vi "moveonapath.vi"() -> ()   [LabVIEW 2017]
uses:
  040-typeDefs/Position.ctl
panel:
  out "Waveform Chart":dbl(graph)
  in  "stop 2":bool
  out "XY Graph":cluster{"X":dbl, "Y":dbl}[](graph)
  in  "Array of Points":T1[](array[typedef])=[{"X Pos"=20.0, "Y Pos"=20.0, "Bearing"=0.0}]
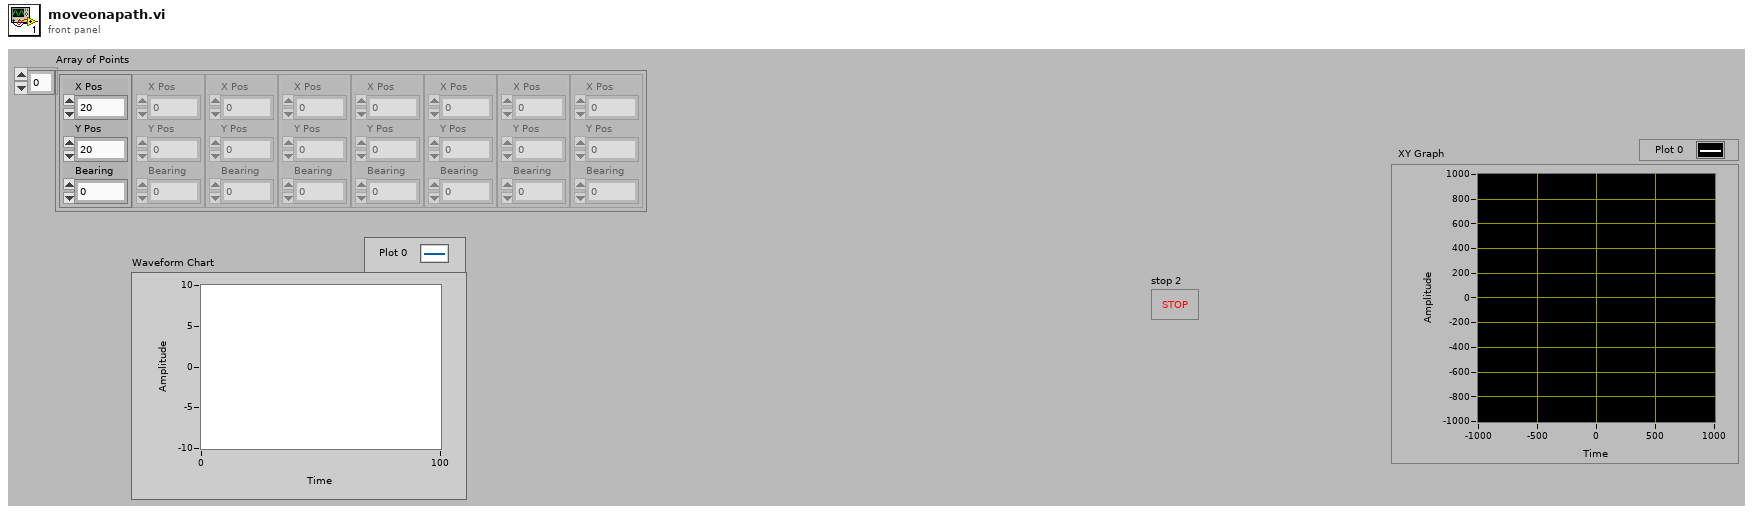
[diagram p1: front panel]
types:
  T1 = typedef "Position.ctl" = cluster{"X Pos":dbl, "Y Pos":dbl, "Bearing":dbl}
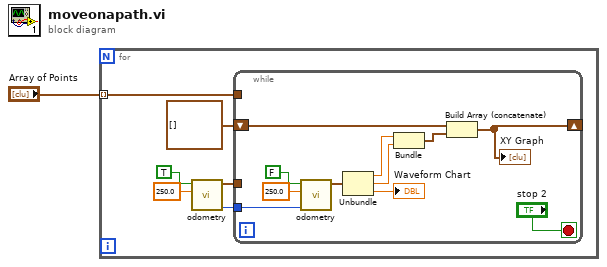
[diagram p0: block diagram]
diagram:
  n1 = for {
    tunnel: "Array of Points" -> [w2] mode=indexing
    n2 = call "odometry.vi"("wheelbase"=250.0, "Position"=TRUE) -> ("ENCB OUT"=w5:i32, "X, Y, BEARING"=w7:cluster{dbl, dbl, dbl})  [unwired: 6 in, 1 out]
    n3 = while {
      tunnel: w7 -> [_]
      shift-right: [w15] -> _
      shift-left: cluster{dbl, dbl}[] [] -> [w16]
      tunnel: w5 -> [w12]
      tunnel: w2 -> [_]
      stop <- "stop 2" stop-if-true
      n4 = call "odometry.vi"("ENCB in"=w12, "wheelbase"=250.0, "Position"=FALSE) -> ("X, Y, BEARING"=w11:cluster{dbl, dbl, dbl})  [unwired: 5 in, 2 out]
      n5 = Unbundle(w11) -> (w18:dbl, w13:dbl, →"Waveform Chart":dbl)
      n6 = Bundle(w18, w13) -> (w17:cluster{dbl, dbl})  [unwired: 1 in]
      n7 = Build Array (concatenate)(w16, w17) -> (w15:cluster{dbl, dbl}[])
      "XY Graph" <- w15
    }
  }
